vi "sub vi - GET ALL TEMP v3.vi"(0 "LA01-EN":bool, 5 "LA02-EN":bool, 7 "LA03-EN":bool, 9 "LA04-EN":bool, 11 "LA05-EN":bool, 12 "Gen Cal Value":dbl) -> (4 "LA01 TEMP":T1, 6 "LA02 TEMP":T1, 8 "LA03 TEMP":T1, 10 "LA04 TEMP":T1, 14 "error":bool, 15 "LA05 TEMP":T1)   [LabVIEW 2013]
panel:
  out "LOOP TIME":dbl
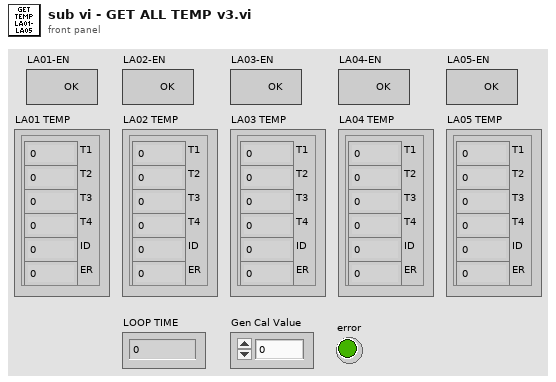
[diagram p1: front panel]
types:
  T1 = cluster{"T1":dbl, "T2":dbl, "T3":dbl, "T4":dbl, "ID":dbl, "ER":dbl}
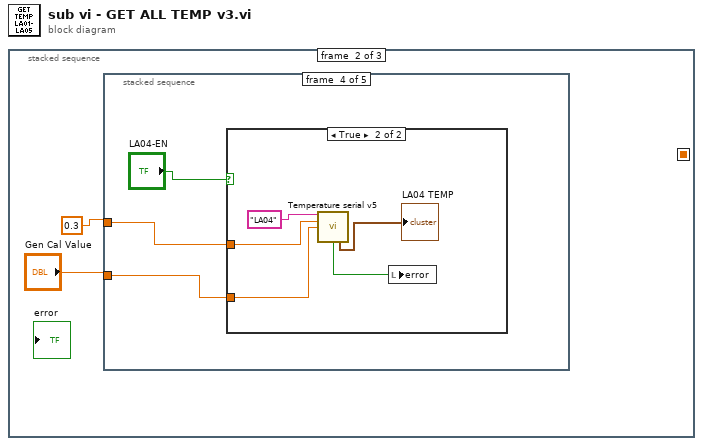
[diagram p0: block diagram]
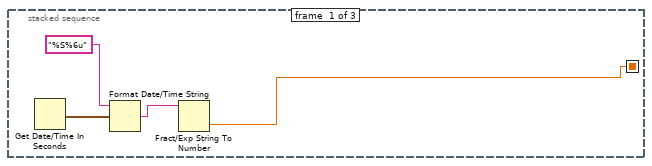
[diagram p2: hidden frame]
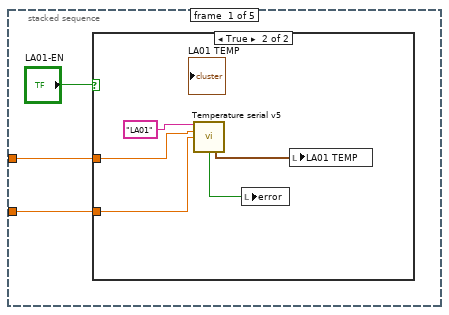
[diagram p3: hidden frame]
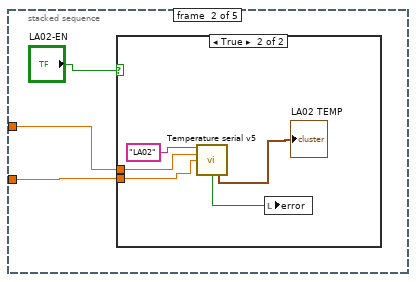
[diagram p5: hidden frame]
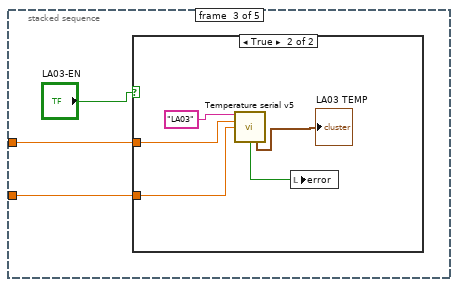
[diagram p7: hidden frame]
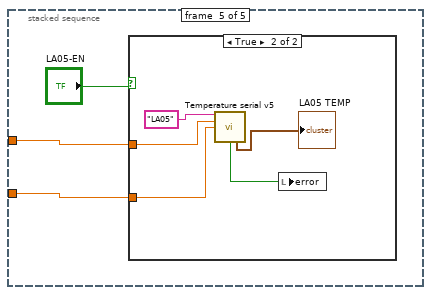
[diagram p10: hidden frame]
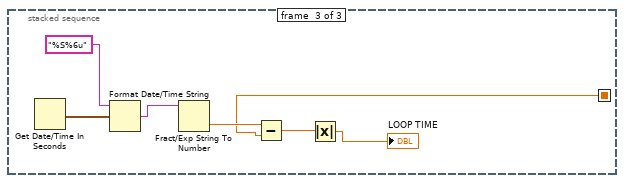
[diagram p12: hidden frame]
diagram:
  n1 = stacked-sequence {
    seq-local: [w1 _ _] -> [_ _ w49]
    frame #0 {
      n2 = Get Date/Time In Seconds() -> (seconds since 1Jan1904=w4:timestamp)
      n3 = Format Date/Time String(time format string (%c)="%S%6u", seconds (now)=w4) -> (date/time string=w2:string)  [unwired: 1 in]
      n4 = Fract/Exp String To Number(string=w2) -> (number=w1:dbl)  [unwired: 3 in, 1 out]
    }
    frame #1 {
      n5 = stacked-sequence {
        tunnel: 0.3 -> [w9 w17 w25 w33 w41]
        tunnel: "Gen Cal Value" -> [w8 w16 w24 w32 w40]
        frame #0 {
          n6 = case shown="True" "LA01-EN" {
            tunnel: w9 -> [_ w13]
            tunnel: w8 -> [_ w12]
            frame False {
            }
            frame True {
              n7 = call "Temperature serial v5.vi"("Command String"="LA01", "Time Out (S)"=w13, "CALIB"=w12) -> ("error"=w11:bool, "output cluster"=w10:cluster{dbl, dbl, dbl, dbl, i32, "error #":dbl})  [unwired: 6 in, 5 out]
              n8 = local write "error"(w11) -> ()
              n9 = local write "LA01 TEMP"(w10) -> ()
            }
          }
        }
        frame #1 {
          n10 = case shown="True" "LA02-EN" {
            tunnel: w17 -> [_ w21]
            tunnel: w16 -> [_ w20]
            frame False {
            }
            frame True {
              n11 = call "Temperature serial v5.vi"("Command String"="LA02", "Time Out (S)"=w21, "CALIB"=w20) -> ("error"=w19:bool, "output cluster"=→"LA02 TEMP":cluster{dbl, dbl, dbl, dbl, i32, "error #":dbl})  [unwired: 6 in, 5 out]
              n12 = local write "error"(w19) -> ()
            }
          }
        }
        frame #2 {
          n13 = case shown="True" "LA03-EN" {
            tunnel: w25 -> [_ w29]
            tunnel: w24 -> [_ w28]
            frame False {
            }
            frame True {
              n14 = call "Temperature serial v5.vi"("Command String"="LA03", "Time Out (S)"=w29, "CALIB"=w28) -> ("error"=w27:bool, "output cluster"=→"LA03 TEMP":cluster{dbl, dbl, dbl, dbl, i32, "error #":dbl})  [unwired: 6 in, 5 out]
              n15 = local write "error"(w27) -> ()
            }
          }
        }
        frame #3 {
          n16 = case shown="True" "LA04-EN" {
            tunnel: w33 -> [_ w37]
            tunnel: w32 -> [_ w36]
            frame False {
            }
            frame True {
              n17 = call "Temperature serial v5.vi"("Command String"="LA04", "Time Out (S)"=w37, "CALIB"=w36) -> ("error"=w35:bool, "output cluster"=→"LA04 TEMP":cluster{dbl, dbl, dbl, dbl, i32, "error #":dbl})  [unwired: 6 in, 5 out]
              n18 = local write "error"(w35) -> ()
            }
          }
        }
        frame #4 {
          n19 = case shown="True" "LA05-EN" {
            tunnel: w41 -> [_ w45]
            tunnel: w40 -> [_ w44]
            frame False {
            }
            frame True {
              n20 = call "Temperature serial v5.vi"("Command String"="LA05", "Time Out (S)"=w45, "CALIB"=w44) -> ("error"=w43:bool, "output cluster"=→"LA05 TEMP":cluster{dbl, dbl, dbl, dbl, i32, "error #":dbl})  [unwired: 6 in, 5 out]
              n21 = local write "error"(w43) -> ()
            }
          }
        }
      }
    }
    frame #2 {
      n22 = Get Date/Time In Seconds() -> (seconds since 1Jan1904=w53:timestamp)
      n23 = Format Date/Time String(time format string (%c)="%S%6u", seconds (now)=w53) -> (date/time string=w51:string)  [unwired: 1 in]
      n24 = Fract/Exp String To Number(string=w51) -> (number=w50:dbl)  [unwired: 3 in, 1 out]
      n25 = Subtract(x=w50, y=w49) -> (x-y=w48:dbl)
      n26 = Absolute Value(x=w48) -> (abs(x)=→"LOOP TIME":dbl)
    }
  }
